vi "Describe Write Error.vi"(7 "Config File Path":path=path "C:/ProgramData/PVI Systems/Staple Inspection System/Config.ini", 8 "error in (no error)":errorcluster, 11 "Mode":T1) -> (0 "error out":errorcluster)   [LabVIEW 2018, in "Config Module.lvlib"]
uses:
  Config Module.lvlib
  Controls/Config File Operation Enum.ctl
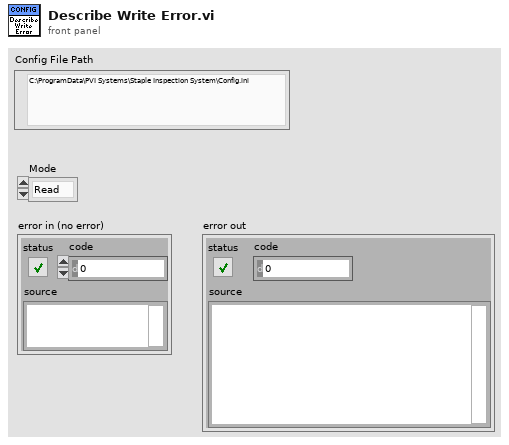
[diagram p1: front panel]
types:
  T1 = typedef "Config Module.lvlib/Config File Operation Enum.ctl" = enum16{"Read", "Write"}
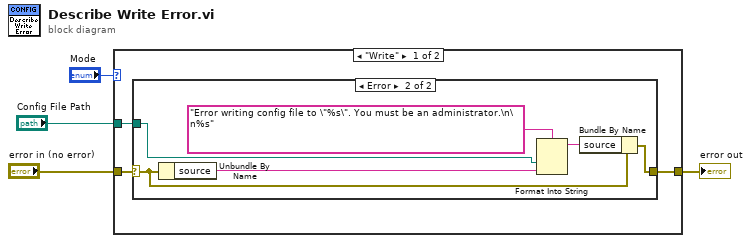
[diagram p0: block diagram]
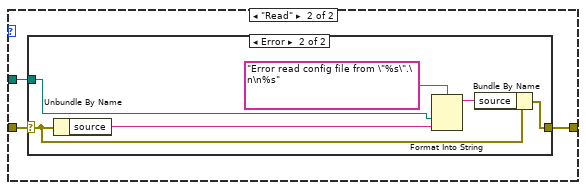
[diagram p3: hidden frame]
diagram:
  n1 = case shown="\"Write\"" "Mode" {
    tunnel: "error in (no error)" -> [w7 w17]
    tunnel: [w6 w16] -> w3
    tunnel: "Config File Path" -> [w5 w15]
    frame "Write" {
      n2 = case shown="Error" w7 {
        selector: w7 -> [w8 w12]
        tunnel: [w8 w9] -> w6
        tunnel: w5 -> [_ w13]
        frame No Error {
        }
        frame Error {
          n3 = Unbundle By Name(w12) -> ("source"=w11:string)
          n4 = Format Into String(format string="Error writing config file to \"%s\". You must be an administrator.\n\n%s", w13, w11) -> (resulting string=w10:string)  [unwired: 2 in, 1 out]
          n5 = Bundle By Name(cluster=w12, "source"=w10) -> (w9:errorcluster)
        }
      }
    }
    frame "Read" {
      n6 = case shown="Error" w17 {
        selector: w17 -> [w18 w22]
        tunnel: [w18 w19] -> w16
        tunnel: w15 -> [_ w23]
        frame No Error {
        }
        frame Error {
          n7 = Unbundle By Name(w22) -> ("source"=w21:string)
          n8 = Format Into String(format string="Error read config file from \"%s\".\n\n%s", w23, w21) -> (resulting string=w20:string)  [unwired: 2 in, 1 out]
          n9 = Bundle By Name(cluster=w22, "source"=w20) -> (w19:errorcluster)
        }
      }
    }
  }
  "error out" <- w3
